vi "Generate Position Setpoints.vi"(10 "Select List":T1(ring)) -> (2 "Targets":T2[](array[typedef]) {"Position" min=-0.5 max=0.5 step=0.1 format="%.2g"})   [LabVIEW 2009]
uses:
  Target.ctl
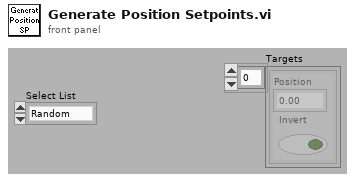
[diagram p1: front panel]
types:
  T1 = enum16{"Random", "List 1", "List 2", "List 3", "List 4", "List 5"}
  T2 = typedef "Target.ctl" = cluster{"Position":dbl, "Invert":bool}
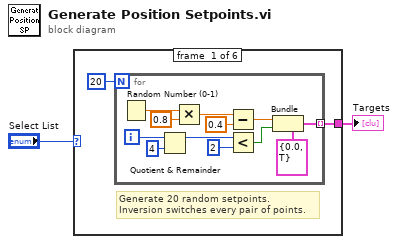
[diagram p0: block diagram]
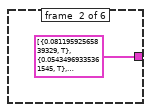
[diagram p2: hidden frame]
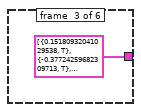
[diagram p3: hidden frame]
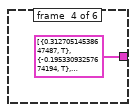
[diagram p4: hidden frame]
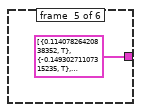
[diagram p5: hidden frame]
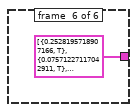
[diagram p6: hidden frame]
diagram:
  n1 = case shown="\"Random\"" "Select List" {
    tunnel: [w4 T2[] [{"Position"=0.08119592565839329, "Invert"=TRUE}, {"Position"=0.05434969335361545, "Invert"=TRUE}, {"Position"=-0.2007431916130365, "Invert"=FALSE}, {"Position"=0.2310713291585873, "Invert"=FALSE}, {"Position"=0.37460234848931084, "Invert"=TRUE}, {"Position"=-0.25592452121687026, "Invert"=TRUE}, {"Position"=0.132152539065453, "Invert"=FALSE}, {"Position"=-0.06835677948542163, "Invert"=FALSE}, {"Position"=0.20487502373709565, "Invert"=TRUE}, {"Position"=-0.12427397542961, "Invert"=TRUE}, {"Position"=-0.031079949293679632, "Invert"=FALSE}, {"Position"=0.13134507601229206, "Invert"=FALSE}, {"Position"=-0.27277113312950796, "Invert"=TRUE}, {"Position"=-0.3740156158503098, "Invert"=TRUE}, {"Position"=0.3931939559040267, "Invert"=FALSE}, {"Position"=-0.27013986488477715, "Invert"=FALSE}, {"Position"=-0.1818266814299758, "Invert"=TRUE}, {"Position"=-0.16058178136584936, "Invert"=TRUE}, {"Position"=0.09167607873989125, "Invert"=FALSE}, {"Position"=0.10463623265464794, "Invert"=FALSE}] ("Targets") T2[] [{"Position"=0.15180932041029538, "Invert"=TRUE}, {"Position"=-0.37724259682309713, "Invert"=TRUE}, {"Position"=-0.36481515692565286, "Invert"=FALSE}, {"Position"=0.39932730597598987, "Invert"=FALSE}, {"Position"=-0.10371556048507974, "Invert"=TRUE}, {"Position"=0.22674810396040002, "Invert"=TRUE}, {"Position"=-0.23885360788792306, "Invert"=FALSE}, {"Position"=-0.08012427890666063, "Invert"=FALSE}, {"Position"=-0.39783777621168537, "Invert"=TRUE}, {"Position"=-0.22236887733375177, "Invert"=TRUE}, {"Position"=-0.34933369028541555, "Invert"=FALSE}, {"Position"=0.23990487962202234, "Invert"=FALSE}, {"Position"=-0.36024139002669353, "Invert"=TRUE}, {"Position"=-0.1644579758575631, "Invert"=TRUE}, {"Position"=0.32257960263922625, "Invert"=FALSE}, {"Position"=0.30610526289560347, "Invert"=FALSE}, {"Position"=0.046490297682885484, "Invert"=TRUE}, {"Position"=0.20003121967076598, "Invert"=TRUE}, {"Position"=-0.24718911428676177, "Invert"=FALSE}, {"Position"=0.201358746316333, "Invert"=FALSE}] ("Targets") T2[] [{"Position"=0.31270514538647487, "Invert"=TRUE}, {"Position"=-0.19533093257674194, "Invert"=TRUE}, {"Position"=-0.053798927427819276, "Invert"=FALSE}, {"Position"=-0.14364408399721923, "Invert"=FALSE}, {"Position"=-0.01602428057703109, "Invert"=TRUE}, {"Position"=-0.26321572562606765, "Invert"=TRUE}, {"Position"=-0.313475923961137, "Invert"=FALSE}, {"Position"=-0.24712200111722105, "Invert"=FALSE}, {"Position"=-0.3953442181911049, "Invert"=TRUE}, {"Position"=-0.1342445700821559, "Invert"=TRUE}, {"Position"=-0.3724224430565123, "Invert"=FALSE}, {"Position"=0.24473920666358928, "Invert"=FALSE}, {"Position"=-0.22743076140072205, "Invert"=TRUE}, {"Position"=0.0031521746969692677, "Invert"=TRUE}, {"Position"=-0.27879657355348936, "Invert"=FALSE}, {"Position"=-0.041945066685094734, "Invert"=FALSE}, {"Position"=0.0747778838514197, "Invert"=TRUE}, {"Position"=-0.15343622336721374, "Invert"=TRUE}, {"Position"=0.21046205700208298, "Invert"=FALSE}, {"Position"=0.10979391290158769, "Invert"=FALSE}] ("Targets") T2[] [{"Position"=0.11407826420838352, "Invert"=TRUE}, {"Position"=-0.14930271107315235, "Invert"=TRUE}, {"Position"=-0.37814800107762725, "Invert"=FALSE}, {"Position"=-0.1733313086588284, "Invert"=FALSE}, {"Position"=0.2525149848785392, "Invert"=TRUE}, {"Position"=0.1779372325293782, "Invert"=TRUE}, {"Position"=-0.1142497157487311, "Invert"=FALSE}, {"Position"=-0.19502403104466615, "Invert"=FALSE}, {"Position"=0.24637317602998554, "Invert"=TRUE}, {"Position"=0.3387583177815333, "Invert"=TRUE}, {"Position"=-0.1209152532261415, "Invert"=FALSE}, {"Position"=0.34839963205968427, "Invert"=FALSE}, {"Position"=0.39609512766519506, "Invert"=TRUE}, {"Position"=-0.21846388379252277, "Invert"=TRUE}, {"Position"=0.1675222716376077, "Invert"=FALSE}, {"Position"=-0.0901295202318394, "Invert"=FALSE}, {"Position"=-0.18267443893911592, "Invert"=TRUE}, {"Position"=0.2888655051513651, "Invert"=TRUE}, {"Position"=-0.05120324654277619, "Invert"=FALSE}, {"Position"=-0.028781501871432247, "Invert"=FALSE}] ("Targets") T2[] [{"Position"=0.2528195718907166, "Invert"=TRUE}, {"Position"=0.07571227117042911, "Invert"=TRUE}, {"Position"=-0.017572258264627605, "Invert"=FALSE}, {"Position"=-0.2741836446068844, "Invert"=FALSE}, {"Position"=-0.39822720129117717, "Invert"=TRUE}, {"Position"=0.05290447392597597, "Invert"=TRUE}, {"Position"=0.03616658235581394, "Invert"=FALSE}, {"Position"=0.1316510758494388, "Invert"=FALSE}, {"Position"=0.2178733310239116, "Invert"=TRUE}, {"Position"=-0.1682144858805401, "Invert"=TRUE}, {"Position"=-0.33308510852593, "Invert"=FALSE}, {"Position"=-0.1914774626806576, "Invert"=FALSE}, {"Position"=-0.09403037934063396, "Invert"=TRUE}, {"Position"=0.08236268002772718, "Invert"=TRUE}, {"Position"=-0.1875104214747454, "Invert"=FALSE}, {"Position"=-0.06978195271943355, "Invert"=FALSE}, {"Position"=0.08569669939089497, "Invert"=TRUE}, {"Position"=0.16707265585848785, "Invert"=TRUE}, {"Position"=-0.33246678953317965, "Invert"=FALSE}, {"Position"=-0.3781577982004805, "Invert"=FALSE}] ("Targets")] -> w2
    frame #0 {
      # "Generate 20 random setpoints.\nInversion switches every pair of points."
      n2 = for {
        N: 20 -> [_]
        tunnel: [w6] -> w4 mode=indexing
        i -> [w12]
        n3 = Random Number (0-1)() -> (number: 0 to 1=w16:dbl)
        n4 = Quotient & Remainder(x=w12, y=4) -> (x-y*floor(x/y)=w10:i32)  [unwired: 1 out]
        n5 = Multiply(x=w16, y=0.8) -> (x*y=w15:dbl)
        n6 = Subtract(x=w15, y=0.4) -> (x-y=w8:dbl)
        n7 = Less?(x=w10, y=2) -> (x < y?=w7:bool)
        n8 = Bundle(cluster=T2 {"Position"=0.0, "Invert"=TRUE} ("Target"), "Position"=w8, "Invert"=w7) -> (w6:T2)
      }
    }
    frame #1 {
    }
    frame #2 {
    }
    frame #3 {
    }
    frame #4 {
    }
    frame #5 {
    }
  }
  "Targets" <- w2
